vi "Status monitoring.vi"() -> ()   [LabVIEW 2014]
uses:
  Golbal Variable/String.vi
panel:
  in  "停止":bool
  out "全局监控":T1
  # "全\n局\n监\n控"
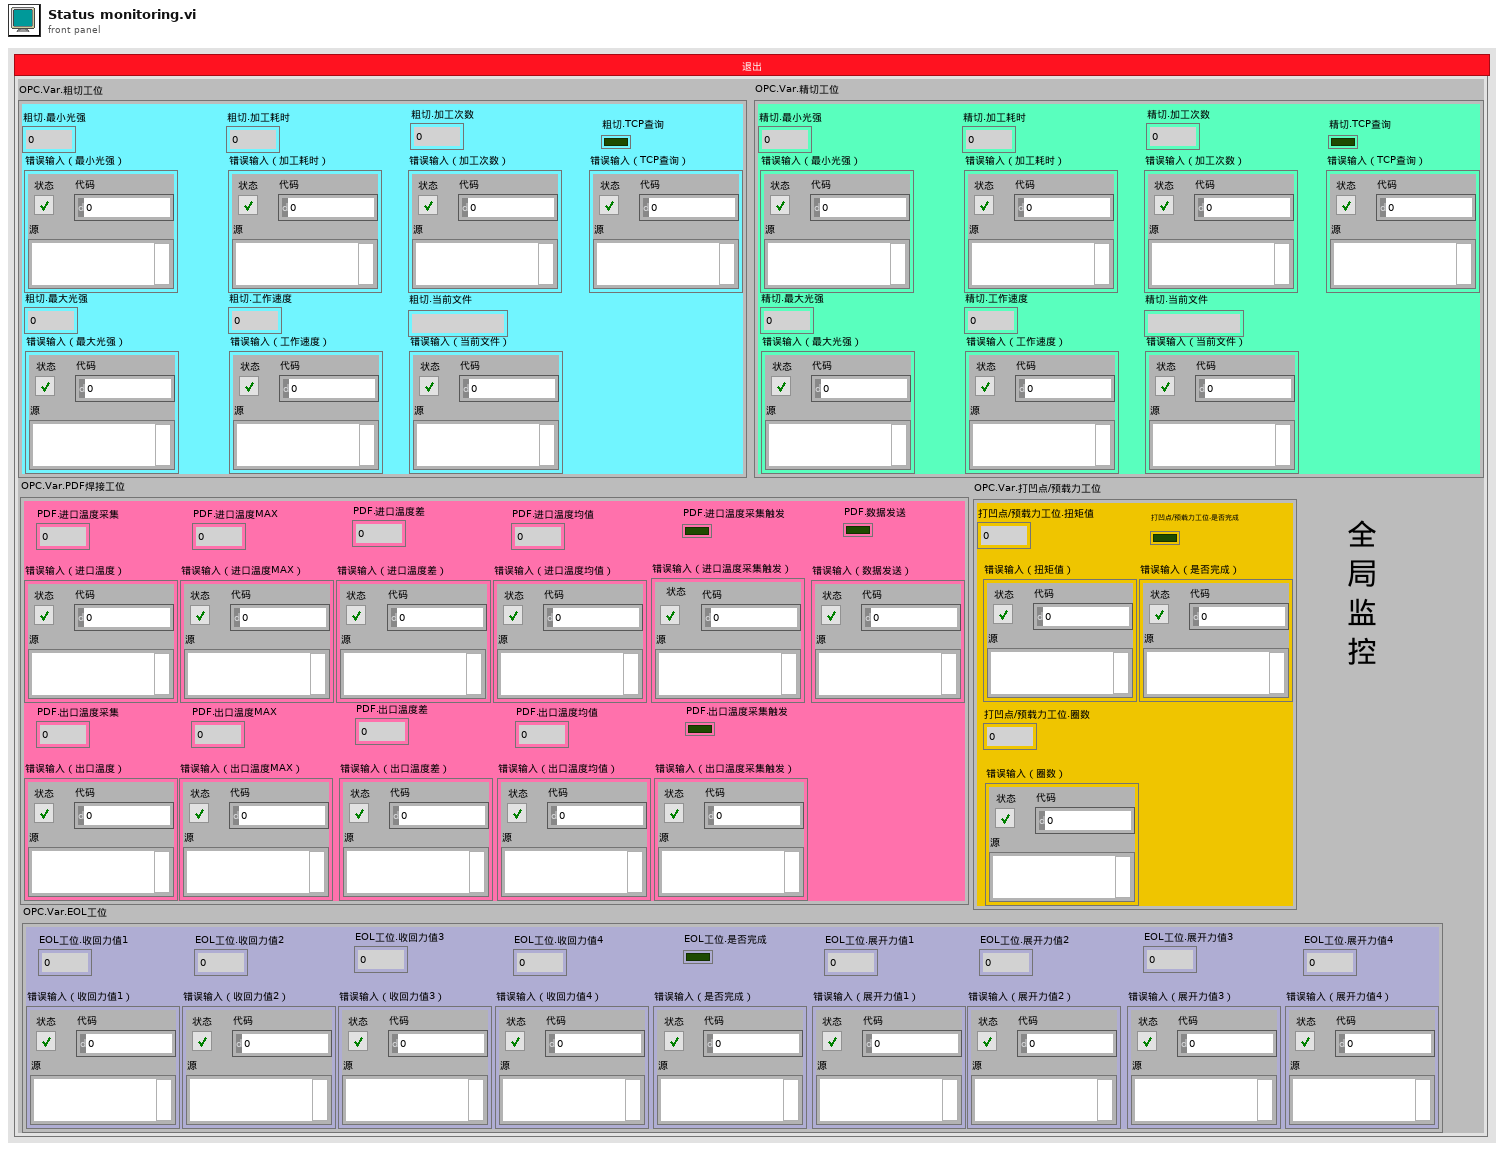
[diagram p1: front panel]
types:
  T1 = cluster{"OPC.Var.粗切工位":cluster{"粗切.最小光强":u16, "error in (no error)":errorcluster, "粗切.最大光强":u16, "error in (no error) 2":errorcluster, "粗切.加工耗时":u16, "error in (no error) 3":errorcluster, "粗切.工作速度":u16, "error in (no error) 4":errorcluster, "粗切.加工次数":u16, "error in (no error) 5":errorcluster, "粗切.当前文件":string, "error in (no error) 6":errorcluster, "粗切.TCP查询":bool, "error in (no error) 7":errorcluster}, "OPC.Var.精切工位":cluster{"精切.最小光强":u16, "error in (no error)":errorcluster, "精切.最大光强":u16, "error in (no error) 2":errorcluster, "精切.加工耗时":u16, "error in (no error) 3":errorcluster, "精切.工作速度":u16, "error in (no error) 4":errorcluster, "精切.加工次数":u16, "error in (no error) 5":errorcluster, "精切.当前文件":string, "error in (no error) 6":errorcluster, "精切.TCP查询":bool, "error in (no error) 7":errorcluster}, "OPC.Var.PDF焊接工位":cluster{"PDF.进口温度采集":u16, "error in (no error)":errorcluster, "PDF.进口温度MAX":u16, "error in (no error) 3":errorcluster, "PDF.进口温度差":u16, "error in (no error) 5":errorcluster, "PDF.进口温度均值":u16, "error in (no error) 7":errorcluster, "PDF.进口温度采集触发":bool, "error in (no error) 8":errorcluster, "PDF.出口温度采集":u16, "error in (no error) 2":errorcluster, "PDF.出口温度MAX":u16, "error in (no error) 4":errorcluster, "PDF.出口温度差":u16, "error in (no error) 6":errorcluster, "PDF.出口温度均值":u16, "error in (no error) 9":errorcluster, "PDF.出口温度采集触发":bool, "error in (no error) 10":errorcluster, "PDF.数据发送":bool, "error in (no error) 11":errorcluster}, "OPC.Var.EOL工位":cluster{"EOL工位.收回力值1":u16, "error in (no error)":errorcluster, "EOL工位.收回力值2":u16, "error in (no error) 3":errorcluster, "EOL工位.收回力值3":u16, "error in (no error) 5":errorcluster, "EOL工位.收回力值4":u16, "error in (no error) 7":errorcluster, "EOL工位.展开力值1":u16, "error in (no error) 2":errorcluster, "EOL工位.展开力值2":u16, "error in (no error) 4":errorcluster, "EOL工位.展开力值3":u16, "error in (no error) 6":errorcluster, "EOL工位.展开力值4":u16, "error in (no error) 9":errorcluster, "EOL工位.是否完成":bool, "error in (no error) 8":errorcluster}, "OPC.Var.打凹点/预载力工位":cluster{"打凹点/预载力工位.扭矩值":u16, "error in (no error)":errorcluster, "打凹点/预载力工位.圈数":u16, "error in (no error) 2":errorcluster, "打凹点/预载力工位.是否完成":bool, "error in (no error) 7":errorcluster}}
  T2 = cluster{"PA10.最小光强":u16, "error in (no error)":errorcluster, "PA10.最大光强":u16, "error in (no error) 2":errorcluster, "PA10.加工耗时":u16, "error in (no error) 3":errorcluster, "PA10.工作速度":u16, "error in (no error) 4":errorcluster, "PA10.加工次数":u16, "error in (no error) 5":errorcluster, "PA10.当前文件":string, "error in (no error) 6":errorcluster, "PA10.TCP查询":bool, "error in (no error) 7":errorcluster}
  T3 = cluster{"PA30.最小光强":u16, "error in (no error)":errorcluster, "PA30.最大光强":u16, "error in (no error) 2":errorcluster, "PA30.加工耗时":u16, "error in (no error) 3":errorcluster, "PA30.工作速度":u16, "error in (no error) 4":errorcluster, "PA30.加工次数":u16, "error in (no error) 5":errorcluster, "PA30.当前文件":string, "error in (no error) 6":errorcluster, "PA30.TCP查询":bool, "error in (no error) 7":errorcluster}
  T4 = cluster{"PA50.进口温度采集":u16, "error in (no error)":errorcluster, "PA50.进口温度MAX":u16, "error in (no error) 3":errorcluster, "PA50.进口温度差":u16, "error in (no error) 5":errorcluster, "PA50.进口温度均值":u16, "error in (no error) 7":errorcluster, "PA50.进口温度采集触发":bool, "error in (no error) 8":errorcluster, "PA50.出口温度采集":u16, "error in (no error) 2":errorcluster, "PA50.出口温度MAX":u16, "error in (no error) 4":errorcluster, "PA50.出口温度差":u16, "error in (no error) 6":errorcluster, "PA50.出口温度均值":u16, "error in (no error) 9":errorcluster, "PA50.出口温度采集触发":bool, "error in (no error) 10":errorcluster, "PA50.数据发送":bool, "error in (no error) 11":errorcluster}
  T5 = cluster{"ST30.收回力值1":u16, "error in (no error)":errorcluster, "ST30.收回力值2":u16, "error in (no error) 3":errorcluster, "ST30.收回力值3":u16, "error in (no error) 5":errorcluster, "ST30.收回力值4":u16, "error in (no error) 7":errorcluster, "ST30.展开力值1":u16, "error in (no error) 2":errorcluster, "ST30.展开力值2":u16, "error in (no error) 4":errorcluster, "ST30.展开力值3":u16, "error in (no error) 6":errorcluster, "ST30.展开力值4":u16, "error in (no error) 9":errorcluster, "ST30.是否完成":bool, "error in (no error) 8":errorcluster}
  T6 = cluster{"ST90.扭矩值":u16, "error in (no error)":errorcluster, "ST90.圈数":u16, "error in (no error) 2":errorcluster, "ST90.是否完成":bool, "error in (no error) 7":errorcluster}
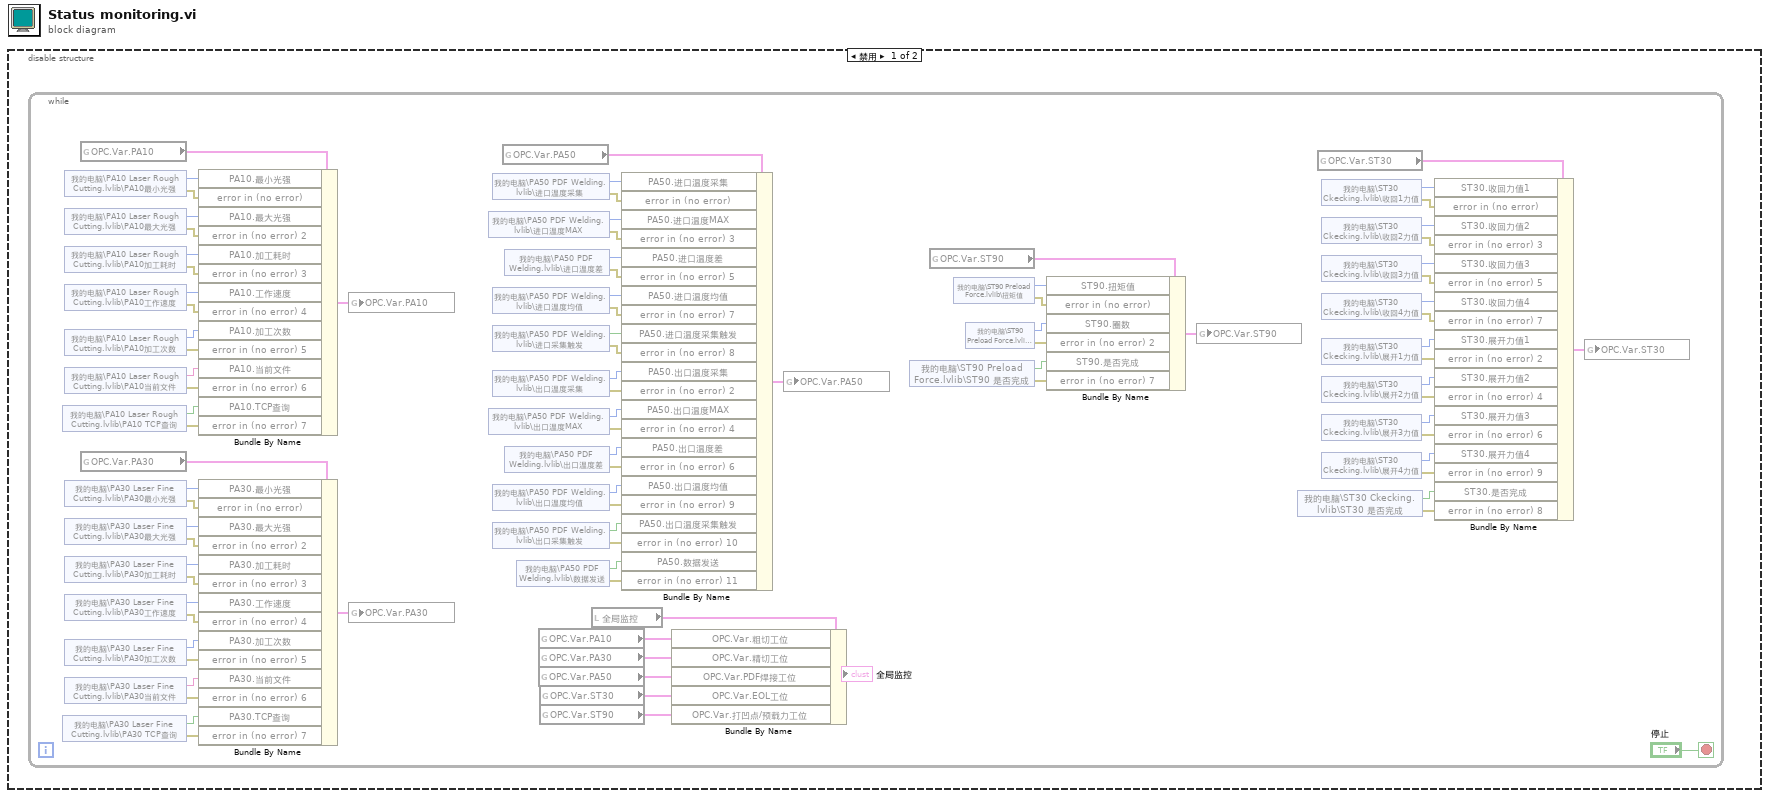
[diagram p0: block diagram]
diagram:
  n1 = disable-structure shown="禁用" {
    frame Disabled {
      n2 = while {
        stop <- "停止" stop-if-true
        n3 = shared-variable "我的电脑\\PA10 Laser Rough Cutting.lvlib\\PA10 TCP查询"() -> (w63:bool, error out=w64:errorcluster)  [unwired: 1 in]
        n4 = shared-variable "我的电脑\\PA30 Laser Fine Cutting.lvlib\\PA30 TCP查询"() -> (w62:bool, error out=w61:errorcluster)  [unwired: 1 in]
        n5 = shared-variable "我的电脑\\PA10 Laser Rough Cutting.lvlib\\PA10最小光强"() -> (w90:u16, error out=w89:errorcluster)  [unwired: 1 in]
        n6 = shared-variable "我的电脑\\PA10 Laser Rough Cutting.lvlib\\PA10最大光强"() -> (w88:u16, error out=w87:errorcluster)  [unwired: 1 in]
        n7 = shared-variable "我的电脑\\PA10 Laser Rough Cutting.lvlib\\PA10加工耗时"() -> (w86:u16, error out=w85:errorcluster)  [unwired: 1 in]
        n8 = shared-variable "我的电脑\\PA10 Laser Rough Cutting.lvlib\\PA10工作速度"() -> (w84:u16, error out=w83:errorcluster)  [unwired: 1 in]
        n9 = shared-variable "我的电脑\\PA10 Laser Rough Cutting.lvlib\\PA10加工次数"() -> (w82:u16, error out=w81:errorcluster)  [unwired: 1 in]
        n10 = shared-variable "我的电脑\\PA10 Laser Rough Cutting.lvlib\\PA10当前文件"() -> (w80:string, error out=w79:errorcluster)  [unwired: 1 in]
        n11 = shared-variable "我的电脑\\PA30 Laser Fine Cutting.lvlib\\PA30最小光强"() -> (w77:u16, error out=w76:errorcluster)  [unwired: 1 in]
        n12 = shared-variable "我的电脑\\PA30 Laser Fine Cutting.lvlib\\PA30最大光强"() -> (w75:u16, error out=w74:errorcluster)  [unwired: 1 in]
        n13 = shared-variable "我的电脑\\PA30 Laser Fine Cutting.lvlib\\PA30加工耗时"() -> (w72:u16, error out=w73:errorcluster)  [unwired: 1 in]
        n14 = shared-variable "我的电脑\\PA30 Laser Fine Cutting.lvlib\\PA30工作速度"() -> (w71:u16, error out=w70:errorcluster)  [unwired: 1 in]
        n15 = shared-variable "我的电脑\\PA30 Laser Fine Cutting.lvlib\\PA30加工次数"() -> (w69:u16, error out=w68:errorcluster)  [unwired: 1 in]
        n16 = shared-variable "我的电脑\\PA30 Laser Fine Cutting.lvlib\\PA30当前文件"() -> (w67:string, error out=w66:errorcluster)  [unwired: 1 in]
        n17 = global read "String.vi" "OPC.Var.PA10"() -> (w92:T2)
        n18 = global read "String.vi" "OPC.Var.PA30"() -> (w78:T3)
        n19 = Bundle By Name(cluster=w92, "PA10.最小光强"=w90, "error in (no error)"=w89, "PA10.最大光强"=w88, "error in (no error) 2"=w87, "PA10.加工耗时"=w86, "error in (no error) 3"=w85, "PA10.工作速度"=w84, "error in (no error) 4"=w83, "PA10.加工次数"=w82, "error in (no error) 5"=w81, "PA10.当前文件"=w80, "error in (no error) 6"=w79, "PA10.TCP查询"=w63, "error in (no error) 7"=w64) -> (w91:T2)
        n20 = Bundle By Name(cluster=w78, "PA30.最小光强"=w77, "error in (no error)"=w76, "PA30.最大光强"=w75, "error in (no error) 2"=w74, "PA30.加工耗时"=w72, "error in (no error) 3"=w73, "PA30.工作速度"=w71, "error in (no error) 4"=w70, "PA30.加工次数"=w69, "error in (no error) 5"=w68, "PA30.当前文件"=w67, "error in (no error) 6"=w66, "PA30.TCP查询"=w62, "error in (no error) 7"=w61) -> (w65:T3)
        n21 = global write "String.vi" "OPC.Var.PA10"(w91) -> ()
        n22 = global write "String.vi" "OPC.Var.PA30"(w65) -> ()
        n23 = shared-variable "我的电脑\\PA50 PDF Welding.lvlib\\进口温度MAX"() -> (w57:i16, error out=w56:errorcluster)  [unwired: 1 in]
        n24 = shared-variable "我的电脑\\PA50 PDF Welding.lvlib\\出口温度MAX"() -> (w47:i16, error out=w46:errorcluster)  [unwired: 1 in]
        n25 = shared-variable "我的电脑\\PA50 PDF Welding.lvlib\\进口温度采集"() -> (w59:u16, error out=w58:errorcluster)  [unwired: 1 in]
        n26 = shared-variable "我的电脑\\PA50 PDF Welding.lvlib\\进口温度均值"() -> (w53:i16, error out=w52:errorcluster)  [unwired: 1 in]
        n27 = shared-variable "我的电脑\\PA50 PDF Welding.lvlib\\进口采集触发"() -> (w51:bool, error out=w50:errorcluster)  [unwired: 1 in]
        n28 = shared-variable "我的电脑\\PA50 PDF Welding.lvlib\\出口温度采集"() -> (w49:u16, error out=w48:errorcluster)  [unwired: 1 in]
        n29 = shared-variable "我的电脑\\PA50 PDF Welding.lvlib\\出口温度均值"() -> (w43:i16, error out=w42:errorcluster)  [unwired: 1 in]
        n30 = shared-variable "我的电脑\\PA50 PDF Welding.lvlib\\出口采集触发"() -> (w41:bool, error out=w40:errorcluster)  [unwired: 1 in]
        n31 = global read "String.vi" "OPC.Var.PA50"() -> (w60:T4)
        n32 = shared-variable "我的电脑\\PA50 PDF Welding.lvlib\\进口温度差"() -> (w55:i16, error out=w54:errorcluster)  [unwired: 1 in]
        n33 = shared-variable "我的电脑\\PA50 PDF Welding.lvlib\\出口温度差"() -> (w45:i16, error out=w44:errorcluster)  [unwired: 1 in]
        n34 = shared-variable "我的电脑\\PA50 PDF Welding.lvlib\\数据发送"() -> (w39:bool, error out=w38:errorcluster)  [unwired: 1 in]
        n35 = global read "String.vi" "OPC.Var.PA10"() -> (w7:T2)
        n36 = global read "String.vi" "OPC.Var.PA30"() -> (w6:T3)
        n37 = global read "String.vi" "OPC.Var.PA50"() -> (w5:T4)
        n38 = global read "String.vi" "OPC.Var.ST30"() -> (w4:T5)
        n39 = global read "String.vi" "OPC.Var.ST90"() -> (w3:T6)
        n40 = local read "全局监控"() -> (w8:T1)
        n41 = Bundle By Name(cluster=w60, "PA50.进口温度采集"=w59, "error in (no error)"=w58, "PA50.进口温度MAX"=w57, "error in (no error) 3"=w56, "PA50.进口温度差"=w55, "error in (no error) 5"=w54, "PA50.进口温度均值"=w53, "error in (no error) 7"=w52, "PA50.进口温度采集触发"=w51, "error in (no error) 8"=w50, "PA50.出口温度采集"=w49, "error in (no error) 2"=w48, "PA50.出口温度MAX"=w47, "error in (no error) 4"=w46, "PA50.出口温度差"=w45, "error in (no error) 6"=w44, "PA50.出口温度均值"=w43, "error in (no error) 9"=w42, "PA50.出口温度采集触发"=w41, "error in (no error) 10"=w40, "PA50.数据发送"=w39, "error in (no error) 11"=w38) -> (w37:T4)
        n42 = Bundle By Name(cluster=w8, "OPC.Var.粗切工位"=w7, "OPC.Var.精切工位"=w6, "OPC.Var.PDF焊接工位"=w5, "OPC.Var.EOL工位"=w4, "OPC.Var.打凹点/预载力工位"=w3) -> (→"全局监控":T1)
        n43 = global write "String.vi" "OPC.Var.PA50"(w37) -> ()
        n44 = shared-variable "我的电脑\\ST90 Preload Force.lvlib\\ST90 是否完成"() -> (w31:bool, error out=w30:errorcluster)  [unwired: 1 in]
        n45 = global read "String.vi" "OPC.Var.ST90"() -> (w36:T6)
        n46 = shared-variable "我的电脑\\ST90 Preload Force.lvlib\\扭矩值"() -> (w35:i32, error out=w34:errorcluster)  [unwired: 1 in]
        n47 = shared-variable "我的电脑\\ST90 Preload Force.lvlib\\圈数"() -> (w33:u16, error out=w32:errorcluster)  [unwired: 1 in]
        n48 = Bundle By Name(cluster=w36, "ST90.扭矩值"=w35, "error in (no error)"=w34, "ST90.圈数"=w33, "error in (no error) 2"=w32, "ST90.是否完成"=w31, "error in (no error) 7"=w30) -> (w29:T6)
        n49 = global write "String.vi" "OPC.Var.ST90"(w29) -> ()
        n50 = shared-variable "我的电脑\\ST30 Ckecking.lvlib\\ST30 是否完成"() -> (w11:bool, error out=w10:errorcluster)  [unwired: 1 in]
        n51 = global read "String.vi" "OPC.Var.ST30"() -> (w28:T5)
        n52 = shared-variable "我的电脑\\ST30 Ckecking.lvlib\\收回1力值"() -> (w27:u32, error out=w26:errorcluster)  [unwired: 1 in]
        n53 = shared-variable "我的电脑\\ST30 Ckecking.lvlib\\收回2力值"() -> (w25:u32, error out=w24:errorcluster)  [unwired: 1 in]
        n54 = shared-variable "我的电脑\\ST30 Ckecking.lvlib\\收回3力值"() -> (w23:u32, error out=w22:errorcluster)  [unwired: 1 in]
        n55 = shared-variable "我的电脑\\ST30 Ckecking.lvlib\\收回4力值"() -> (w21:u32, error out=w20:errorcluster)  [unwired: 1 in]
        n56 = shared-variable "我的电脑\\ST30 Ckecking.lvlib\\展开1力值"() -> (w19:u32, error out=w18:errorcluster)  [unwired: 1 in]
        n57 = shared-variable "我的电脑\\ST30 Ckecking.lvlib\\展开2力值"() -> (w17:u32, error out=w16:errorcluster)  [unwired: 1 in]
        n58 = shared-variable "我的电脑\\ST30 Ckecking.lvlib\\展开3力值"() -> (w15:u32, error out=w14:errorcluster)  [unwired: 1 in]
        n59 = shared-variable "我的电脑\\ST30 Ckecking.lvlib\\展开4力值"() -> (w13:u32, error out=w12:errorcluster)  [unwired: 1 in]
        n60 = Bundle By Name(cluster=w28, "ST30.收回力值1"=w27, "error in (no error)"=w26, "ST30.收回力值2"=w25, "error in (no error) 3"=w24, "ST30.收回力值3"=w23, "error in (no error) 5"=w22, "ST30.收回力值4"=w21, "error in (no error) 7"=w20, "ST30.展开力值1"=w19, "error in (no error) 2"=w18, "ST30.展开力值2"=w17, "error in (no error) 4"=w16, "ST30.展开力值3"=w15, "error in (no error) 6"=w14, "ST30.展开力值4"=w13, "error in (no error) 9"=w12, "ST30.是否完成"=w11, "error in (no error) 8"=w10) -> (w9:T5)
        n61 = global write "String.vi" "OPC.Var.ST30"(w9) -> ()
      }
    }
    frame Enabled {
    }
  }
